vi "queryLaserStatus.vi"(8 "error in (no error)":errorcluster, 11 "CommandCreator in":refnum<class "CommandCreator.lvclass">) -> (0 "error out":errorcluster, 2 "command":string, 3 "CommandCreator out":refnum<class "CommandCreator.lvclass">)   [LabVIEW 2016, in "CommandCreator.lvclass"]
uses:
  CommandCreator.lvclass
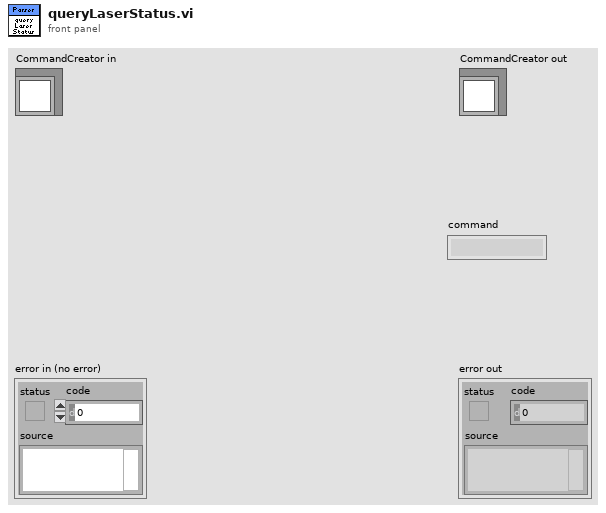
[diagram p1: front panel]
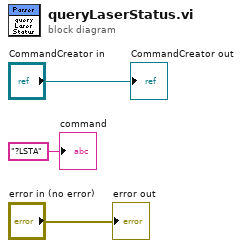
[diagram p0: block diagram]
diagram:
  "error out" <- "error in (no error)"
  "CommandCreator out" <- "CommandCreator in"
  "command" <- "?LSTA" ("command")
